vi "run.vi"(8 "error in (no error)":errorcluster, 9 "?":bool, 10 "Exposure Time (s)":dbl=0.004 min=0.0 step=0.001 format="%.3f", 11 "Camera Handle":u32) -> (0 "error out":errorcluster, 1 "?":u16[](graph), 3 "Camera Handle 2":u32, 7 "PyLoN Ready":bool)   [LabVIEW 2014]
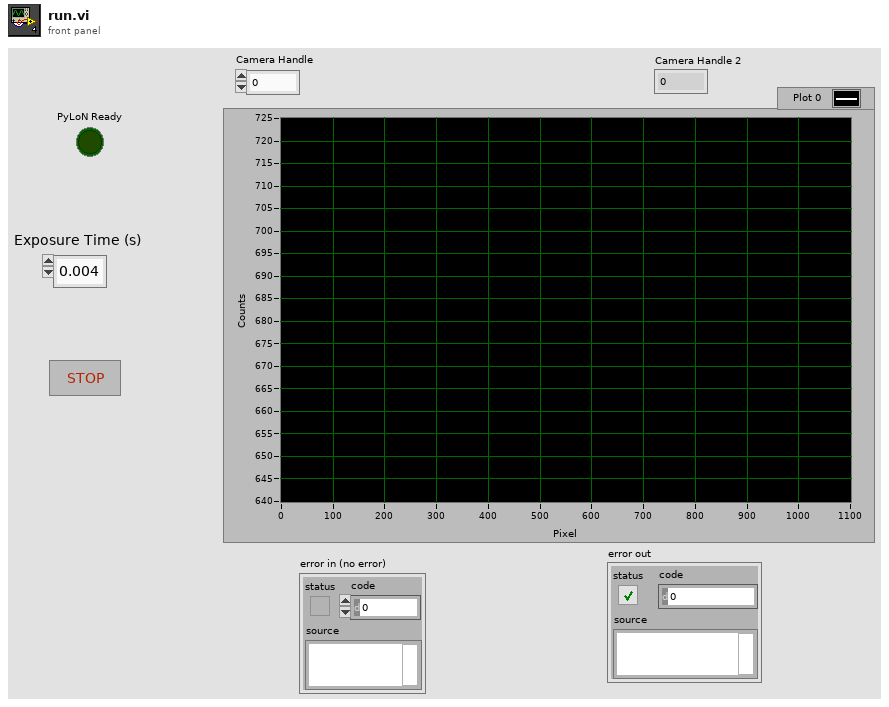
[diagram p1: front panel]
types:
  T1 = cluster{"acquire focus mode":u32, "Exposure Time (s)":dbl, i32, "Software accumulation":u32}
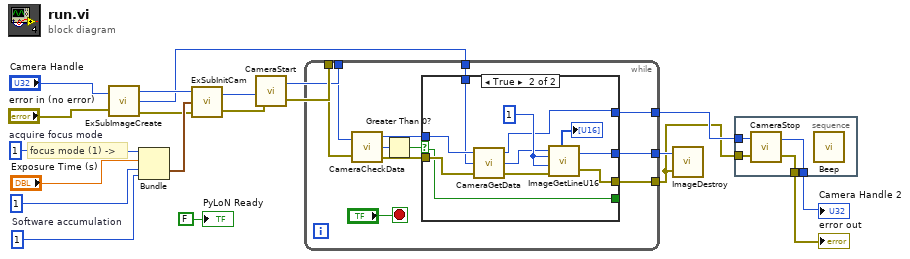
[diagram p0: block diagram]
diagram:
  w19 = u32 1  # acquire focus mode
  w18 = u32 1  # Software accumulation
  # "focus mode (1) ->"
  n1 = call "ExSubImageCreate.vi"("Camera Handle"="Camera Handle", "error in (no error)"="error in (no error)") -> ("Camera Handle"=w17:u32, "Data Handle"=w11:u32, "error out"=w16:errorcluster)
  n2 = Bundle("acquire focus mode"=w19, "Exposure Time (s)"="Exposure Time (s)", 1, "Software accumulation"=w18) -> (w20:T1)  [unwired: 1 in]
  n3 = call "ExSubInitCam.vi"("error in (no error)"=w16, "Camera Information"=w20, "Camera Handle"=w17) -> ("error out"=w15:errorcluster, "Camera Handle"=w14:u32)
  n4 = call <userlib>:"CameraStart.vi"("error in"=w15, "Camera Handle"=w14) -> ("error out"=w13:errorcluster, "Camera Handle"=w12:u32)
  n5 = while {
    tunnel: [w26] -> w10
    tunnel: [w25] -> w8
    tunnel: [w24] -> w9
    tunnel: w13 -> [w23]
    tunnel: w12 -> [w22]
    tunnel: w11 -> [w21]
    stop <- "?" stop-if-true
    n6 = call <userlib>:"CameraCheckData.vi"("Camera Handle"=w22, "error in"=w23) -> ("Camera Handle"=w29:u32, "Number Of Frames Available"=w31:i32, "error out"=w28:errorcluster)
    n7 = Greater Than 0?(x=w31) -> (x > 0?=w30:bool)
    n8 = case shown="True" w30 {
      selector: w30 -> [w34 w44]
      tunnel: w29 -> [w32 w46]
      tunnel: w28 -> [w35 w45]
      tunnel: [w34 w44] -> _
      tunnel: [w35 w42] -> w25
      tunnel: w21 -> [w33 w36]
      tunnel: [w33 w40] -> w26
      tunnel: [w32 w39] -> w24
      frame False {
      }
      frame True {
        w41 = 1
        n9 = call <userlib>:"CameraGetData.vi"("error in"=w45, "Data Handle"=w36, "Camera Handle"=w46) -> ("error out"=w38:errorcluster, "Data Handle"=w37:u32, "Camera Handle"=w39:u32)
        n10 = call <userlib>:"ImageGetLineU16.vi"("Data Handle"=w37, "Y Position"=w41, "Z Position"=w41, "error in"=w38) -> ("Array u16"=→"?":u16[], "Data Handle"=w40:u32, "error out"=w42:errorcluster)
      }
    }
  }
  n11 = call <userlib>:"ImageDestroy.vi"("error in"=w8, "Data handle"=w10) -> ()  [unwired: 1 out]
  n12 = stacked-sequence {
    tunnel: w8 -> [w50]
    tunnel: w9 -> [w49]
    tunnel: [w48] -> w2
    tunnel: [w47] -> w3
    frame #0 {
      n13 = call <userlib>:"CameraStop.vi"("error in"=w50, "Camera Handle"=w49) -> ("error out"=w48:errorcluster, "Camera Handle"=w47:u32)
      n14 = call <vilib>:"Beep.vi"() -> ()  [unwired: 12 in]
    }
  }
  "Camera Handle 2" <- w3
  "error out" <- w2
  "PyLoN Ready" <- FALSE ("PyLoN Ready")
